vi "Configure test.vi"(6 "Assert VI Path":path, 7 "Existing Queue Elements":string, 8 "error in (no error)":errorcluster, 11 "FP LT in":refnum<class "FP LT.lvclass">) -> (0 "error out":errorcluster, 3 "FP LT out":refnum<class "FP LT.lvclass">)   [LabVIEW 2018, in "FP LT.lvclass"]
uses:
  FP LT.lvclass
  3ee150a4-778f-43bd-adbd-e60bf9bd1af6.vi
  <vilib>/JDP Science/JSONtext/Find Item.vi
  3ee150a4-778f-43bd-adbd-e60bf9bd1af6.vi/2d1d15b2-290b-4484-8500-1305f3584b0b.vi
  3ee150a4-778f-43bd-adbd-e60bf9bd1af6.vi/cfab416e-aa8b-4a4e-a407-b751ba6573e6.vi
  <vilib>/JDP Science/JSONtext/String Subset.vi
  Test Class String IDs.vi
  <vilib>/JDP Science/JSONtext/Parsing/Parse Full Path or Item Name.vi
  <vilib>/JDP Science/JSONtext/Offset/Find Item Locations by Path.vi
  <vilib>/JDP Science/JSONtext/JSON text to Variant.vi
  <vilib>/JDP Science/JSONtext/Variant to JSON Text.vi
  <vilib>/JDP Science/JSONtext/Set Item.vi
  Floating Point.lvclass
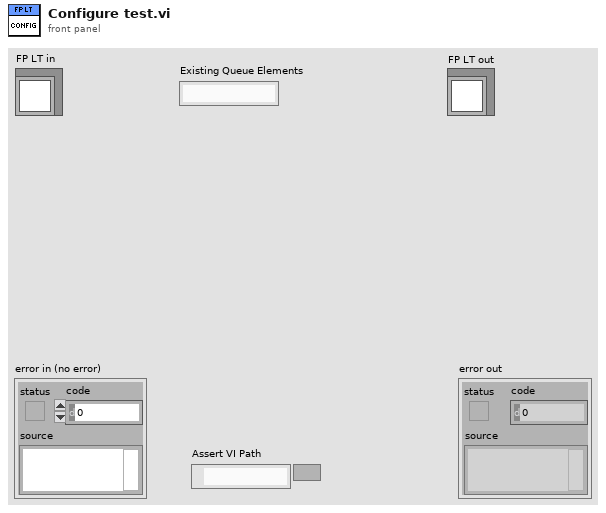
[diagram p1: front panel]
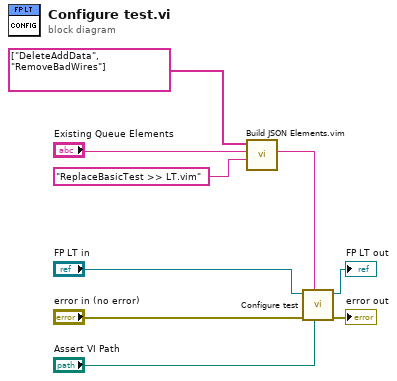
[diagram p0: block diagram]
diagram:
  n1 = call "Build JSON Elements.vim"("Append Element(s)"="ReplaceBasicTest >> LT.vim", "JSON Elements in ({})"="Existing Queue Elements", "Prepend Element(s)"=string[] ["DeleteAddData", "RemoveBadWires"]) -> ("JSON Elements out"=w2:string)  [unwired: 8 in]
  n2 = call-parent "Configure test.vi"("Assert VI Path"="Assert VI Path", "Existing Queue Elements"=w2, "error in (no error)"="error in (no error)", "Floating Point in"="FP LT in") -> ("error out"=→"error out":errorcluster, "Floating Point out"=→"FP LT out":refnum<class "FP LT.lvclass">)  [unwired: 6 in]
